vi "TRAJECTORY_INPUT_SENSORS.vi"(6 "Right Speed":dbl, 7 "Left Distance":dbl, 8 "Left Speed":dbl, 9 "Gyro Continous\n (inc counterclockwise)":dbl, 11 "Right Distance":dbl) -> (3 "Input Sensors":T1)   [LabVIEW 2019]
uses:
  TRAJ_EXEC_INPUT_SENSORS.ctl
  <vilib>/Rock Robotics/WPI/ThirdParty/JAS_Junk/TrajLib/Rotation_CreateAngle.vi
  <vilib>/Rock Robotics/WPI/ThirdParty/JAS_Junk/TrajLib/Translation_Create.vi
  <vilib>/Rock Robotics/WPI/ThirdParty/JAS_Junk/TrajLib/Pose_RelativeTo.vi
  <vilib>/Rock Robotics/WPI/ThirdParty/JAS_Junk/TrajLib/Transform_Create_TransRot.vi
  <vilib>/Rock Robotics/WPI/ThirdParty/JAS_Junk/TrajLib/Transform_Create_PosePose.vi
  <vilib>/Rock Robotics/WPI/ThirdParty/JAS_Junk/TrajLib/Pose_New_TRRO.vi
  <vilib>/Rock Robotics/WPI/ThirdParty/JAS_Junk/TrajLib/Rotation_UnaryMinus.vi
  <vilib>/Rock Robotics/WPI/ThirdParty/JAS_Junk/TrajLib/Translation_RotateBy.vi
  <vilib>/Rock Robotics/WPI/ThirdParty/JAS_Junk/TrajLib/Translation_Minus.vi
  <vilib>/Rock Robotics/WPI/ThirdParty/JAS_Junk/TrajLib/Rotation_Minus.vi
  <vilib>/Rock Robotics/WPI/ThirdParty/JAS_Junk/TrajLib/Rotation_RotateBy.vi
  <vilib>/Rock Robotics/WPI/ThirdParty/JAS_Junk/TrajLib/Rotation_CreateXY.vi
  <vilib>/Rock Robotics/WPI/ThirdParty/JAS_Junk/TrajLib/Util_CalcDist.vi
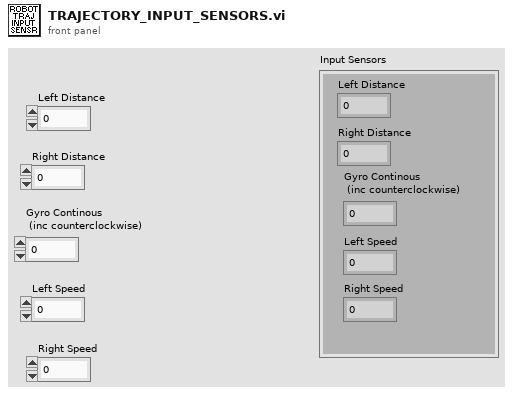
[diagram p1: front panel]
types:
  T1 = typedef "TRAJ_EXEC_INPUT_SENSORS.ctl" = cluster{"Left Distance":dbl, "Right Distance":dbl, "Gyro Continous\n (inc counterclockwise)":dbl, "Left Speed":dbl, "Right Speed":dbl}
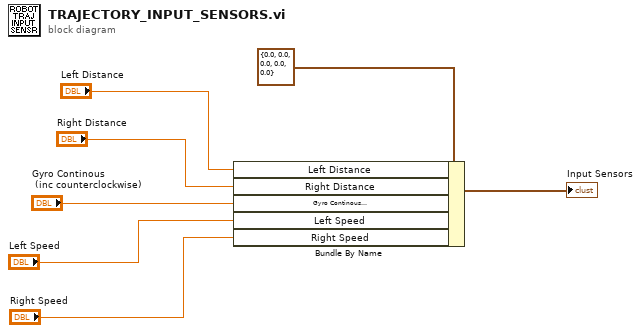
[diagram p0: block diagram]
diagram:
  n1 = Bundle By Name(cluster=T1 {"Left Distance"=0.0, "Right Distance"=0.0, "Gyro Continous\n (inc counterclockwise)"=0.0, "Left Speed"=0.0, "Right Speed"=0.0} ("Input Sensors 2"), "Left Distance"="Left Distance", "Right Distance"="Right Distance", "Gyro Continous\n (inc counterclockwise)"="Gyro Continous\n (inc counterclockwise)", "Left Speed"="Left Speed", "Right Speed"="Right Speed") -> (→"Input Sensors":T1)
